vi "Validate connectio to osc.vi"(8 "error in (no error)":errorcluster, 11 "Datos Osciloscopio":T1 {"Número Promedio" min=2 max=20}) -> (0 "error out":errorcluster, 2 "Success?":bool)   [LabVIEW 2020]
uses:
  Type Definitions/datos osciloscopio.ctl
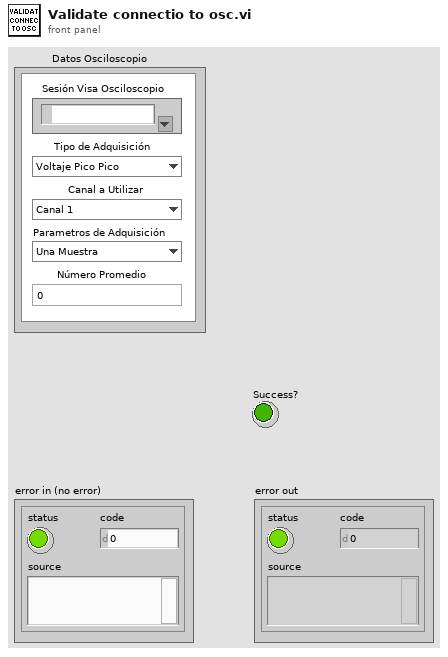
[diagram p1: front panel]
types:
  T1 = typedef "datos osciloscopio.ctl" = cluster{"Sesión Visa Osciloscopio":refnum<visa-resource-name>, "Tipo de Adquisición":enum16{"Voltaje Pico Pico", "Voltaje RMS", "Cursor Tiempo"}, "Canal a Utilizar":enum16{"Canal 1", "Canal 2", "Canal 1 y 2"}, "Parametros de Adquisición":enum16{"Una Muestra", "Promedio"}, "Número Promedio":i32}
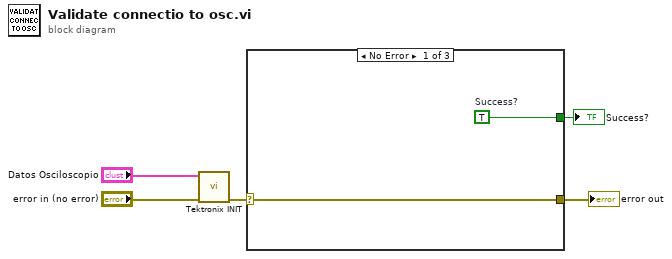
[diagram p0: block diagram]
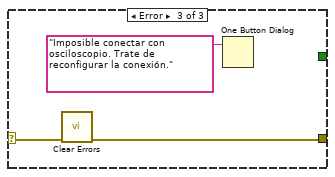
[diagram p3: hidden frame]
diagram:
  n1 = call "Tektronix INIT.vi"("error in (no error)"="error in (no error)", "Datos Osciloscopio"="Datos Osciloscopio") -> ("error out"=w3:errorcluster)  [unwired: 9 in]
  n2 = case shown="No Error" w3 {
    selector: w3 -> [w7 w8 w11]
    tunnel: [w7 w8 w10] -> w2
    tunnel: [w6 _ _] -> w1
    frame No Error {
      w6 = TRUE  # Success?
    }
    frame Default {
    }
    frame Error {
      n3 = call <vilib>:"Clear Errors.vi"("error in (no error)"=w11) -> ("error out"=w10:errorcluster)  [unwired: 5 in, 1 out]
      n4 = One Button Dialog(message="Imposible conectar con osciloscopio. Trate de reconfigurar la conexión.") -> ()  [unwired: 1 in, 1 out]
    }
  }
  "error out" <- w2
  "Success?" <- w1
